vi "Configure AI Timing.vi"(8 "error in (no error)":errorcluster, 11 "Task in":refnum<k21>) -> (0 "error out":errorcluster, 2 "AI Timing Settings":string, 3 "Task out":refnum<k21>)   [LabVIEW 2021, in "Load Frame.lvlib"]
uses:
  Load Frame.lvlib
  <vilib>/DAQmx/configure/timing.llb/DAQmx Timing (Sample Clock).vi
  <resource>/objmgr/daqmx.rc
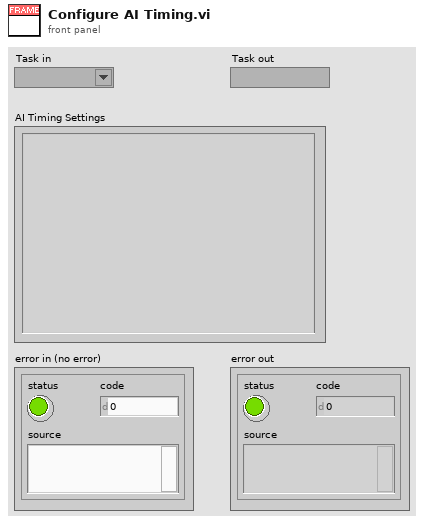
[diagram p1: front panel]
types:
  T1 = cluster{"SampClk.Rate":dbl, "SampClk.MaxRate":dbl}
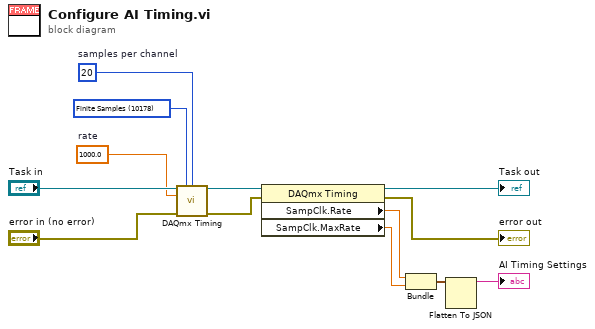
[diagram p0: block diagram]
diagram:
  w7 = 1000.0  # rate
  w6 = 20  # samples per channel
  w5 = 10178 items=["Finite Samples"=10178, "Continuous Samples"=10123, "Hardware Timed Single Point"=12522] ("sample mode")
  n1 = call-poly <vilib>:"DAQmx Timing.vi"("task/channels in"="Task in", "sample mode"=w5, "samples per channel"=w6, "rate"=w7, "error in"="error in (no error)") -> ("task out"=w12:refnum<k21>, "error out"=w10:errorcluster)  [unwired: 9 in]
  n2 = property class="DAQmx Timing"(reference=w12, error in=w10) -> (reference out=→"Task out":refnum<k21>, error out=→"error out":errorcluster, "SampClk.Rate"=w4:dbl, "SampClk.MaxRate"=w3:dbl)
  n3 = Bundle("SampClk.Rate"=w4, "SampClk.MaxRate"=w3) -> (w1:T1)  [unwired: 1 in]
  n4 = Flatten To JSON(anything=w1) -> (JSON string=→"AI Timing Settings":string)  [unwired: 2 in, 1 out]
